vi "Get All Connections.vi"(11 "Route Manager in":refnum<class "SLSC Switch.lvclass">) -> (2 "connections":T1[](array[typedef]), 3 "Route Manager out":refnum<class "SLSC Switch.lvclass">)   [LabVIEW 2016, in "SLSC Switch.lvlib" / "SLSC Switch.lvclass"]
uses:
  SLSC Switch.lvclass
  Controls/Connection.ctl
  SLSC Switch.lvclass/SLSC Switch.ctl
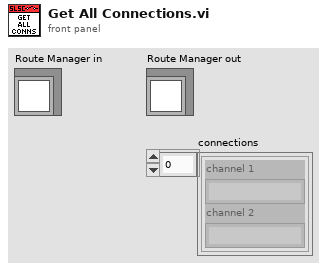
[diagram p1: front panel]
types:
  T1 = typedef "SLSC Switch.lvlib/SLSC Switch.lvclass/Connection.ctl" = cluster{"channel 1":string, "channel 2":string}
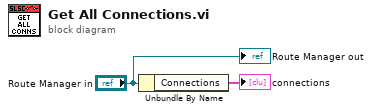
[diagram p0: block diagram]
diagram:
  n1 = Unbundle By Name("Route Manager in") -> ("Connections"=→"connections":T1[])
  "Route Manager out" <- "Route Manager in"
